vi "Day 1.2 - Top Three Calories Total.vi"(11 "input":u64[](array[numeric])) -> (3 "output":u64)   [LabVIEW 2021]
uses:
  9f43e3ef-74e0-4cc9-b794-cc5f2f062fc9.vi
  <vilib>/Comparison/Less/Less Functor/Less Functor.lvclass
panel:
  out "subarray":u64[](array[numeric])
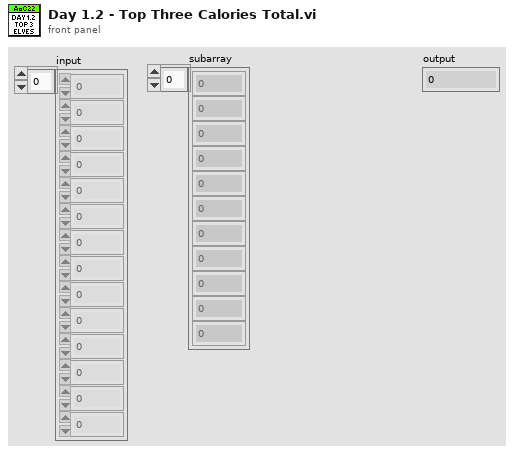
[diagram p1: front panel]
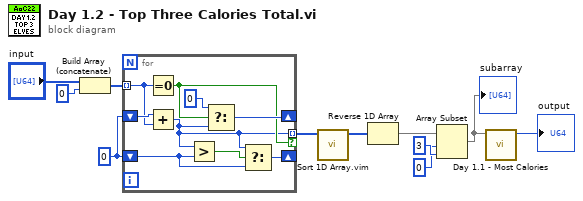
[diagram p0: block diagram]
diagram:
  w10 = u64 0
  n1 = Build Array (concatenate)("input", u64 0) -> (w5:u64[])
  n2 = for {
    tunnel: w5 -> [w19] mode=indexing
    shift-right: [w18] -> _
    shift-left: w10 -> [w20]
    shift-right: [w14] -> _
    shift-left: w10 -> [w15]
    tunnel: [w12] -> w9 mode=indexing if=w13
    n3 = Equal To 0?(x=w19) -> (x = 0?=w13:bool)
    n4 = Add(x=w20, y=w19) -> (x+y=w12:u64)
    n5 = Greater?(x=w12, y=w15) -> (0:w16:bool)
    n6 = Select(t=0, s=w13, f=w12) -> (s? t:f=w18:u64)
    n7 = Select(t=w12, s=w16, f=w15) -> (s? t:f=w14:u64)
  }
  n8 = call "Sort 1D Array.vim"("unsorted array"=w9) -> ("sorted array"=w4:u64[])  [unwired: 10 in]
  n9 = Reverse 1D Array(array=w4) -> (reversed array=w3:u64[])
  n10 = Array Subset(array=w3, index=u64 0 ("new element/subarray"), length=3 ("index")) -> (w8:u64[])
  "subarray" <- w8
  n11 = call "Day 1.1 - Most Calories.vi"("input"=w8) -> ("output"=→"output":u64)  [unwired: 10 in]
